vi "End-Less Array.vi"(11 "Array":dbl[](array[numeric])) -> (3 "Array Without Endpoints":dbl[](array[numeric]))   [LabVIEW 2017]
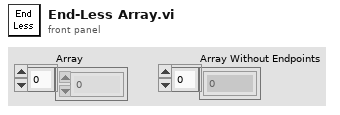
[diagram p1: front panel]
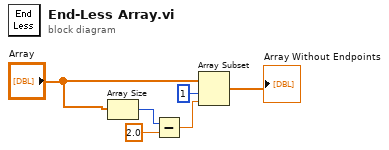
[diagram p0: block diagram]
diagram:
  n1 = Array Size(array="Array") -> (size(s)=w3:i32)
  n2 = Subtract(x=w3, y=2.0) -> (x-y=w4:dbl)
  n3 = Array Subset(array="Array", index=1, length=w4) -> (→"Array Without Endpoints":dbl[])
